vi "Teleop.vi"(10 "Match Info":T1={"Autonomous Elapsed Seconds"=0.0, "TeleOp Elapsed Seconds"=768.189, "Disabled Elapsed Seconds"=20.969, "Visited Autonomous"=FALSE, "Visited TeleOp"=TRUE, "Visited Disabled"=TRUE, "Autonomous Settings"={"Autonomous Style"=enum."Independent", "VI Refnum"=refnum}}, 11 "Call Context":T2=enum."Stop") -> ()   [LabVIEW 2020]
doc: "This VI is called for each TeleOp packet received from the DS where the robot is not disabled. It is often used to read from the joysticks and update I/O or to update setpoints for timed control loops. It should complete and return within 20 milliseconds or it may miss DS packets."
uses:
  <vilib>/Rock Robotics/WPI/DriverStation/WPI_DriverStationDerivedRobotMode.ctl
  <vilib>/Rock Robotics/WPI/DriverStation/WPI_DriverStationMatch Info.ctl
  <vilib>/Rock Robotics/Network Tables/NT Read Boolean.vi
  <vilib>/Rock Robotics/WPI/Utilities/WPI_GetSetVariantRefNum.vi
  <vilib>/Rock Robotics/Network Tables/NT Write Numeric Array.vi
  <vilib>/Rock Robotics/Network Tables/NT Write Boolean Array.vi
  <vilib>/Rock Robotics/Network Tables/NT Write Boolean.vi
  <vilib>/Rock Robotics/Network Tables/NT Read Number.vi
  Robot Global Data.vi
  <vilib>/Rock Robotics/WPI/ThirdParty/Phoenix-LabVIEW/Motor Controller/Controls/CTRE_Phoenix_MotorControl_ControlMode.ctl
  <vilib>/Rock Robotics/Network Tables/NT Write Number.vi
panel:
  out "Sample Boolean 0":bool
  out "Sample Slider 0":dbl(slide) scale=0.0..5.0
  out "Sample Boolean 2":bool
  out "Sample Slider 2":dbl(slide) scale=0.0..5.0
  out "Sample Boolean 1":bool
  out "Sample Slider1":dbl(slide) scale=0.0..5.0
  in  "Joysticks":u16(ring) items=["RIGHT TANK (default)", "LEFT ARM", "RIGHT ARM", "LEFT TANK DRIVE"]
  in  "AXIS VALUES":u16(ring) items=["X axis", "Y axis", "Z axis"]
  in  "NORMAL":cluster{"button":i32, "%speed":dbl}={"button"=0, "%speed"=0.75} {"%speed" min=0.0 max=1.0 format="%.3g"}
  in  "TURTLE":cluster{"button":i32, "%speed":dbl}={"button"=4, "%speed"=0.5} {"%speed" min=0.0 max=1.0 format="%.3g"}
  in  "TURBO":cluster{"button":i32, "%speed":dbl}={"button"=2, "%speed"=1.0} {"%speed" min=0.0 max=1.0 format="%.3g"}
  # "JOYSTICK 1  (left drive)\nBUTTONS & CONTROLS\n\nBTN 0 - BUMP INTAKE \nBTN 1 - FORCE INTAKE down\nBTN 2 -  \nBTN 3 - \nBTN 4 - \nBTN 5 - \nBTN 6 - \n\nPOV - \n\nX - \nY - drive LEFT forward/reverse\nZ -\nROT -"
  # "JOYSTICK 0  (right drive)\nBUTTONS & CONTROLS\n\nBTN 0 - FIRE cargo\nBTN 1 - TURBO drive \nBTN 2 - \nBTN 3 - \nBTN 4 - \nBTN 5 - TURTLE drive\nBTN 6 - RE-CENTER POV camera\n\nPOV - camera servo?\n\nX - drive left/right\nY - drive RIGHT forward/reverse\nZ -\nROT -"
  # "JOYSTICK LEFT  arm\nBUTTONS & CONTROLS\n\nX - left rotate arm forward\nY - forward raises climber\n\nBTN  7 - OVERIDE PGM\nBTN  8 - MACRO FWD\nBTN  9 - MACRO REV \nBTN 10 - TOGGLE INTAKE UP/DN\nBTN 11 - INTAKE ROLLER TOGGLE\nBTN 12 - LOW CLIMB MACRO"
  # "JOYSTICK RIGHT  arm\nBUTTONS & CONTROLS\n\nX - left rotate arm forward\nY - forward raises climber\n\nBTN  7 - FIRE CARGO\nBTN  8 - SHOOTER HI speed\nBTN  9 - SHOOTER LO speed\nBTN 10 - \nBTN 11 - PUKE BALL\nBTN 12 - SHOOTER STOP"
  # "to START MOKEY BAR CLIMBING MACRO, PRESS & HOLD BTN 8 & 9"
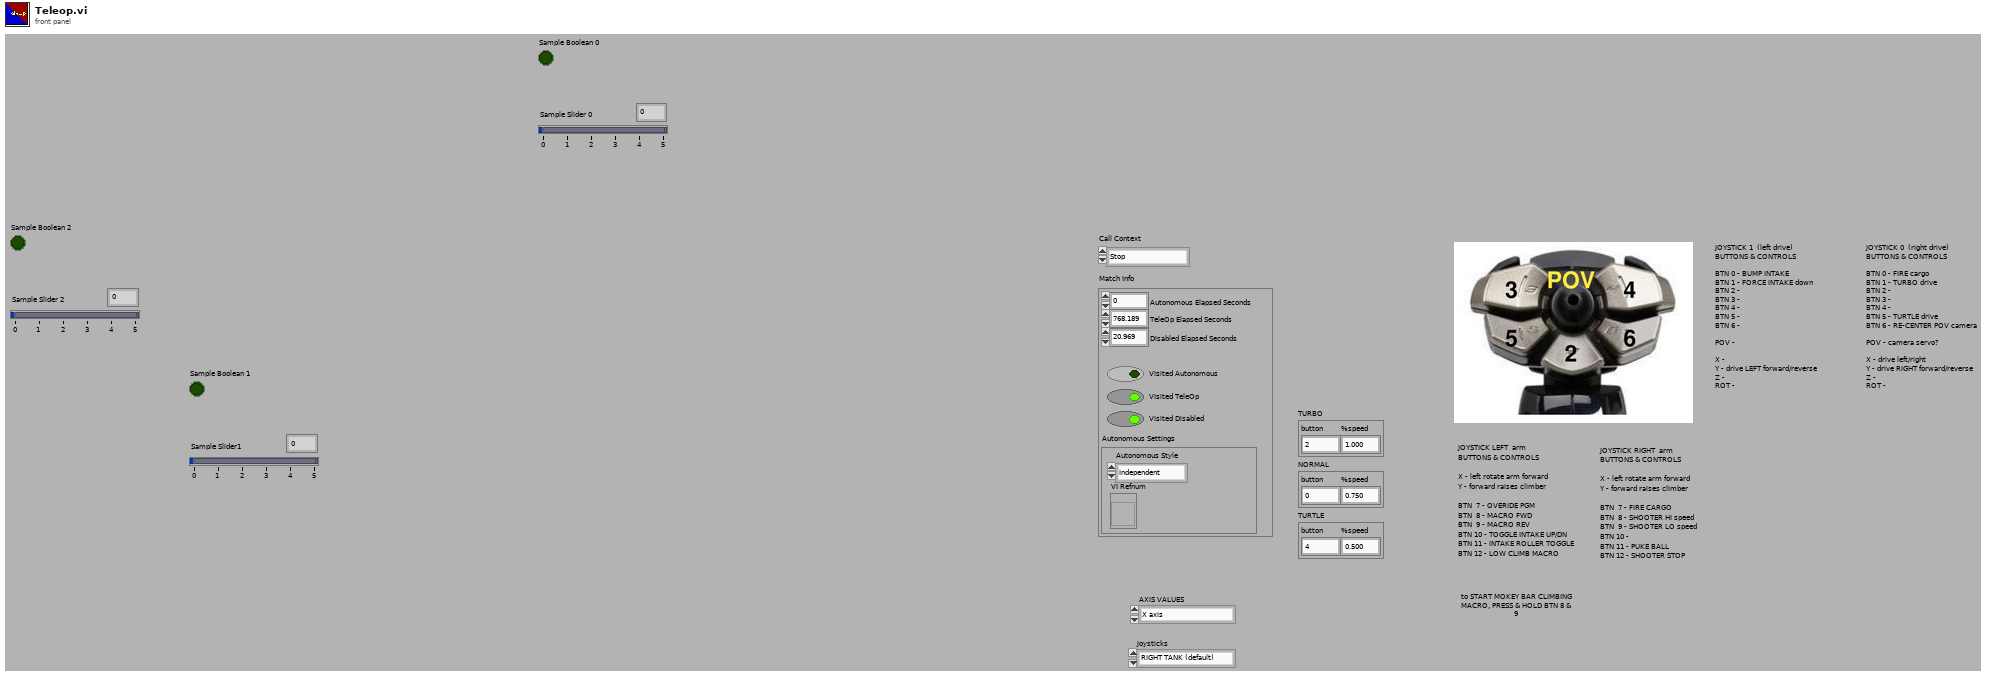
[diagram p1: front panel]
types:
  T1 = typedef "WPI_DriverStationMatch Info.ctl" = cluster{"Autonomous Elapsed Seconds":dbl, "TeleOp Elapsed Seconds":dbl, "Disabled Elapsed Seconds":dbl, "Visited Autonomous":bool, "Visited TeleOp":bool, "Visited Disabled":bool, "Autonomous Settings":cluster{"Autonomous Style":enum16{"Iterative", "Independent"}, "VI Refnum":refnum<vi>}}
  T2 = typedef "WPI_DriverStationDerivedRobotMode.ctl" = enum16{"Init", "Execute", "Stop"}
  T3 = typedef "CTRE_Phoenix_MotorControl_ControlMode.ctl" = u16
  T4 = typedef "WPI_MotorControlDeviceRef.ctl" = cluster{"DeviceStatus":errorcluster, "Type":T5, "PWM":cluster{"PWM Channel":T6, "DeadBand":T7}, "CAN":cluster{"Device Number":u8, "SetOutput VI Ref":variant, "GetOutput VI Ref":variant, "Enable VI Ref":variant, "Disable VI Ref":variant, "Data":variant}, "Invert":bool, "DIO PWM":cluster{"PWM \"Enable\" Channel":T6, "DIOChannel":T8, "PWM Rate":dbl}}
  T5 = typedef "WPI_MotorControlType.ctl" = enum16{"PWM", "CAN", "DIO PWM"}
  T6 = typedef "FPGA_DIOPWMChannel.ctl" = enum8{"PWM 0", "PWM 1", "PWM 2", "PWM 3", "PWM 4", "PWM 5", "PWM 6", "PWM 7", "PWM 8", "PWM 9", "PWM MXP 0", "PWM MXP 1", "PWM MXP 2", "PWM MXP 3", "PWM MXP 4", "PWM MXP 5", "PWM MXP 6", "PWM MXP 7", "PWM MXP 8", "PWM MXP 9", "Invalid"}
  T7 = typedef "WPI_PWMDeadband.ctl" = cluster{"Name":string, "maxPositivePwm":i32, "minPositivePwm":i32, "centerPwm":i32, "maxNegativePwm":i32, "minNegativePwm":i32, "angularRange":u16}
  T8 = typedef "FPGA_DIOChannel.ctl" = enum8{"DIO 0", "DIO 1", "DIO 2", "DIO 3", "DIO 4", "DIO 5", "DIO 6", "DIO 7", "DIO 8", "DIO 9", "DIO MXP 0", "DIO MXP 1", "DIO MXP 2", "DIO MXP 3", "DIO MXP 4", "DIO MXP 5", "DIO MXP 6", "DIO MXP 7", "DIO MXP 8", "DIO MXP 9", "DIO MXP 10", "DIO MXP 11", "DIO MXP 12", "DIO MXP 13", "DIO MXP 14", "DIO MXP 15", "SPI Port CS1", "SPI Port CS2", "SPI Port CS3", "SPI Port MISO", "SPI Port MOSI", "Invalid"}
  T9 = cluster{"MIN":dbl, "MAX":dbl, "convert climber inches to tics":dbl, "INITIALIZE":dbl}
  T10 = typedef "WPI_JoystickDevRef.ctl" = cluster{"Device":T11}
  T11 = typedef "WPI_JoystickDeviceEnum.ctl" = enum16{"USB 0", "USB 1", "USB 2", "USB 3", "USB 4", "USB 5"}
  T12 = cluster{"Axes":dbl[], "Buttons":bool[], "POVs":i16[]}[]
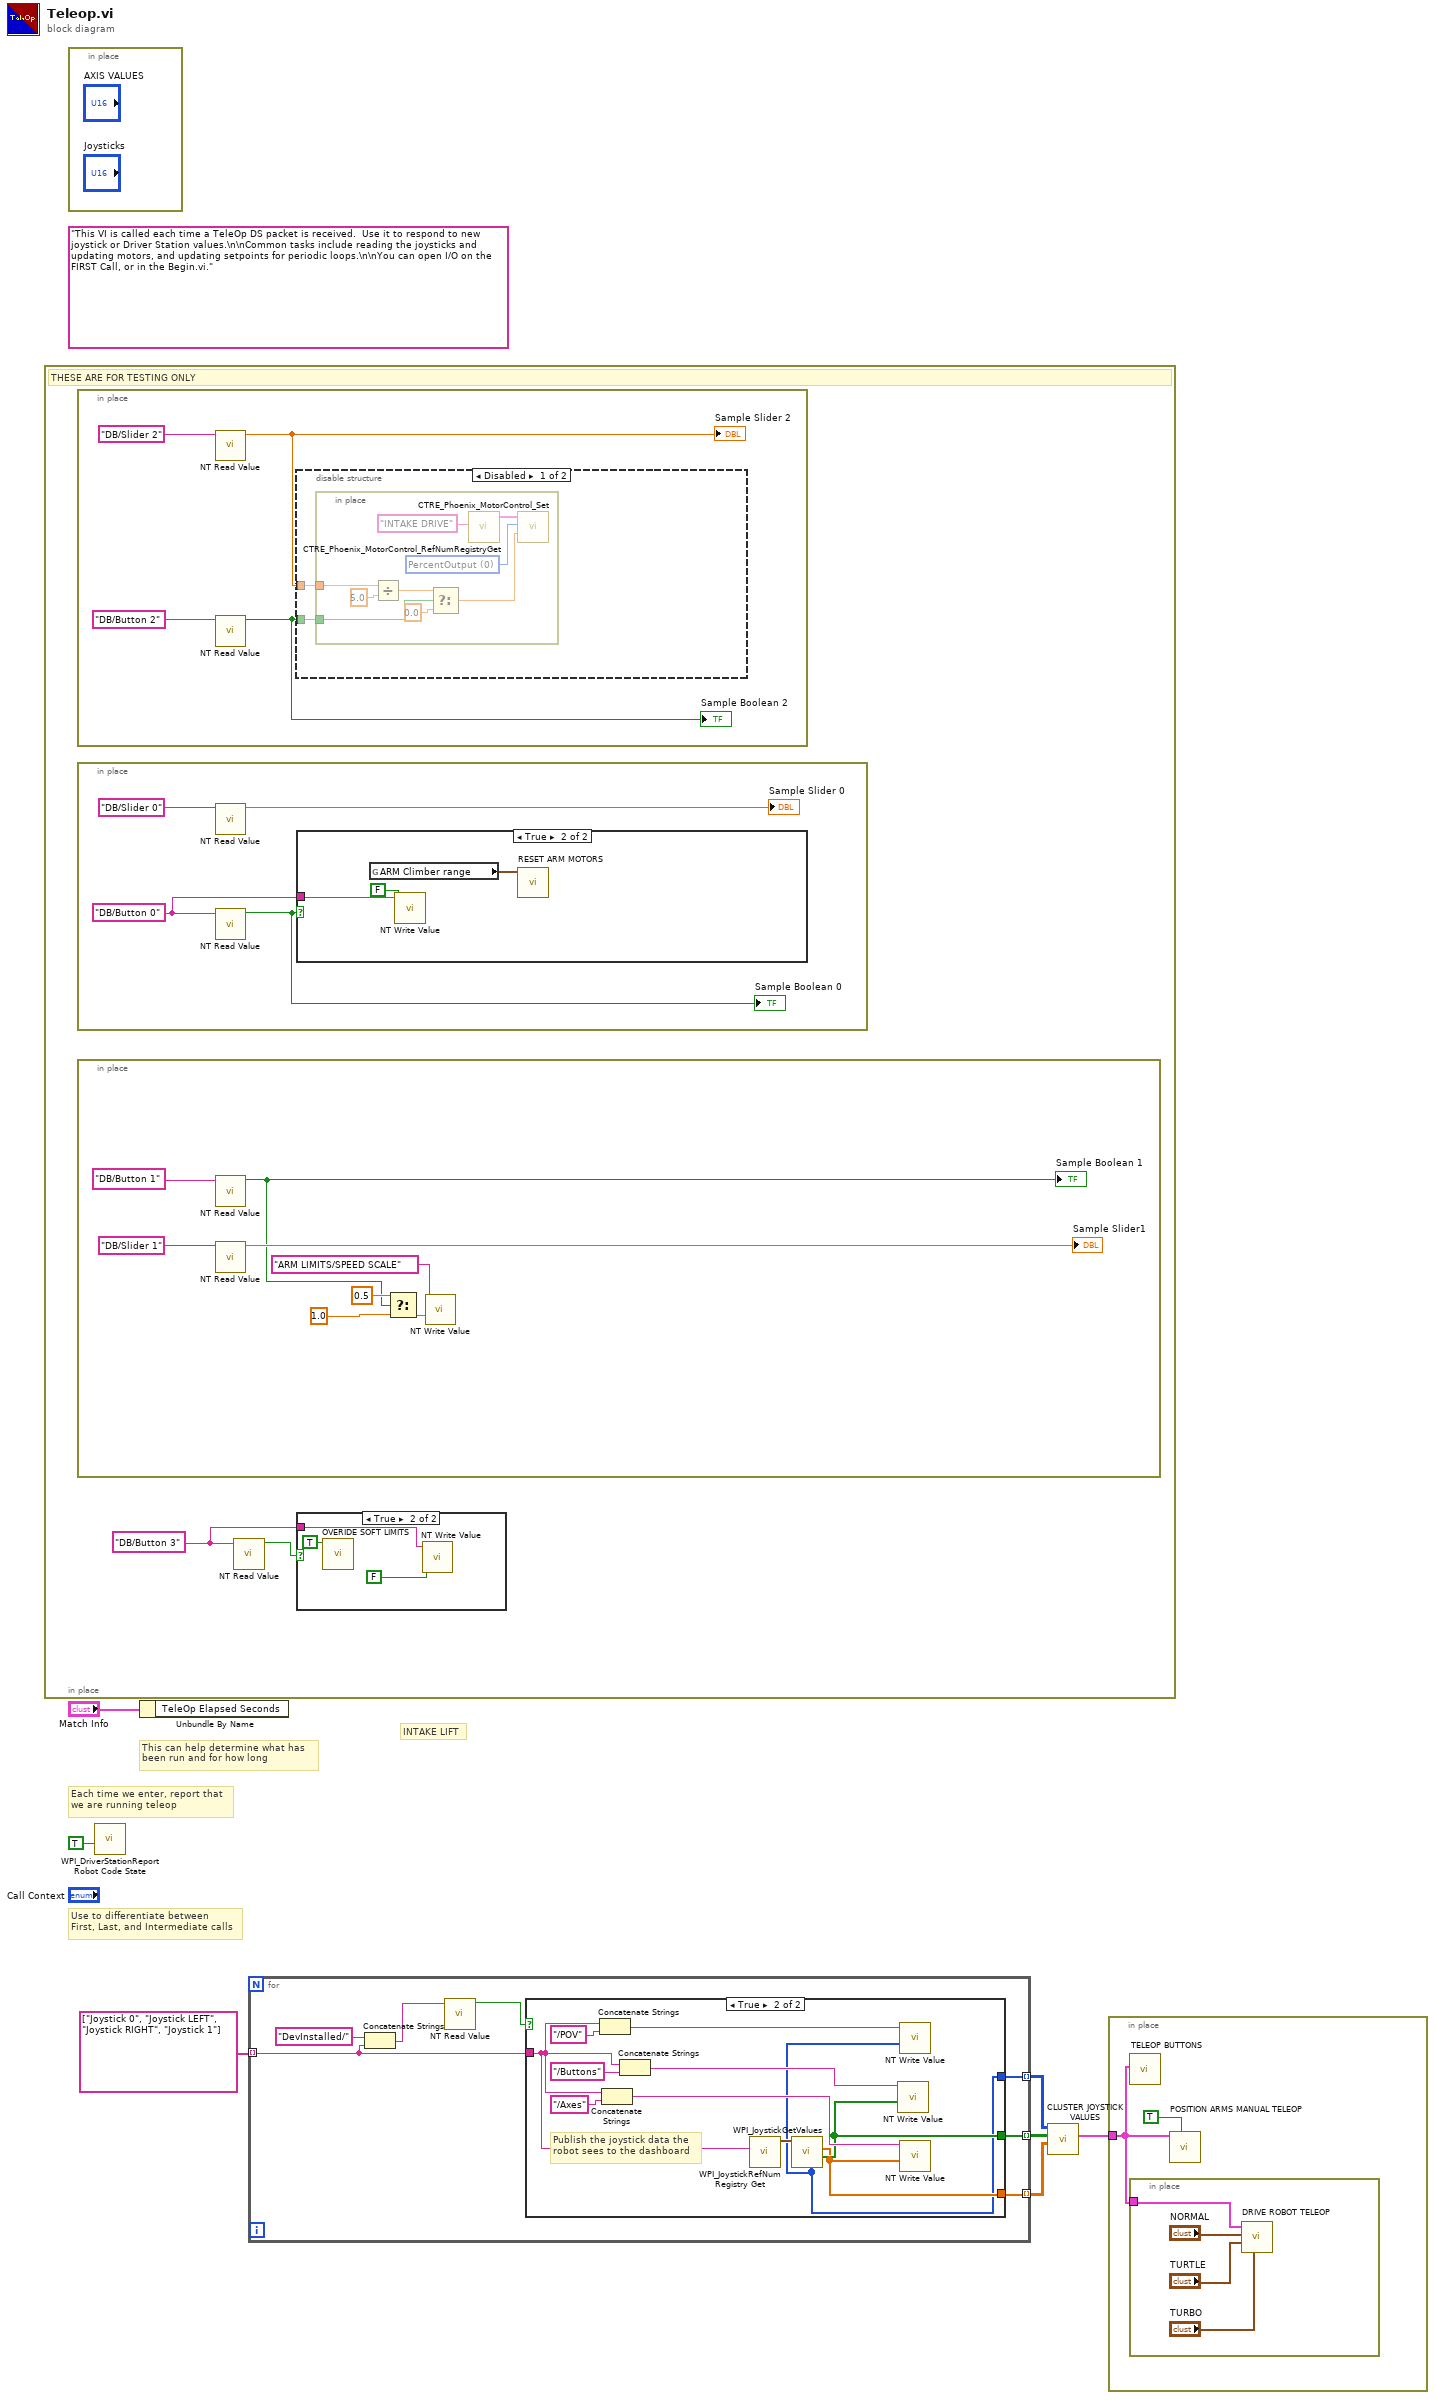
[diagram p0: block diagram]
diagram:
  (unwired) "This VI is called each time a TeleOp DS packet is received.  Use it to respond to new joystick or Driver Station values.\n\nCommon tasks include reading the joysticks and updating motors, and updating setpoints for periodic loops.\n\nYou can open I/O on the FIRST Call, or in the Begin.vi."
  # "INTAKE LIFT"
  # "Each time we enter, report that\nwe are running teleop"
  # "Use to differentiate between\nFirst, Last, and Intermediate calls"
  # "This can help determine what has\nbeen run and for how long"
  n1 = in-place {
    w8 = "DB/Button 3" ("refnum name")
    # "THESE ARE FOR TESTING ONLY"
    n2 = in-place {
      n3 = call-poly <vilib>:"NT Read Value.vi"("Name"="DB/Slider 2" ("refnum name")) -> ("Numeric"=w21:dbl)  [unwired: 9 in, 1 out]
      "Sample Slider 2" <- w21
      n4 = call-poly <vilib>:"NT Read Value.vi"("Name"="DB/Button 2" ("refnum name")) -> ("Boolean"=w20:bool)  [unwired: 9 in, 1 out]
      "Sample Boolean 2" <- w20
      n5 = disable-structure shown="Disabled" {
        disable-tunnel: w21 -> [w25 _]
        disable-tunnel: w20 -> [w24 _]
        frame Disabled {
          n6 = in-place {
            in-place-border: w25 -> [w34]
            in-place-border: w24 -> [w28]
            w31 = T3 0 items=["PercentOutput"=0, "Position"=1, "Velocity"=2, "Current"=3, "Follower"=5, "MotionProfile"=6, "MotionMagic"=7, "MotionProfileArc"=10, "Disabled"=15] ("Control Mode")
            n7 = Divide(x=w34, y=5.0) -> (x/y=w27:dbl)
            n8 = Select(t=w27, s=w28, f=0.0) -> (s? t:f=w29:dbl)
            n9 = call <vilib>:"CTRE_Phoenix_MotorControl_RefNumRegistryGet.vi"("refnum name"="INTAKE DRIVE") -> ("PhoenixMotorControlDevRef"=w32:T4)  [unwired: 9 in, 1 out]
            n10 = call <vilib>:"CTRE_Phoenix_MotorControl_Set.vi"("Output"=w29, "Control Mode"=w31, "PhoenixMotorControlDevRef"=w32) -> ()  [unwired: 7 in, 2 out]
          }
        }
        frame Enabled {
        }
      }
    }
    n11 = in-place {
      w13 = "DB/Button 0" ("refnum name")
      n12 = call-poly <vilib>:"NT Read Value.vi"("Name"="DB/Slider 0" ("refnum name")) -> ("Numeric"=→"Sample Slider 0":dbl)  [unwired: 9 in, 1 out]
      n13 = call-poly <vilib>:"NT Read Value.vi"("Name"=w13) -> ("Boolean"=w14:bool)  [unwired: 9 in, 1 out]
      "Sample Boolean 0" <- w14
      n14 = case shown="True" w14 {
        tunnel: w13 -> [_ w19]
        frame False {
        }
        frame True {
          n15 = global read "Robot Global Data.vi" "ARM Climber range"() -> (w18:T9)
          n16 = call-poly <vilib>:"NT Write Value.vi"("Boolean"=FALSE, "Name"=w19) -> ()  [unwired: 9 in, 1 out]
          n17 = call "RESET ARM MOTORS.vi"("ARM Climber range"=w18) -> ()  [unwired: 8 in, 3 out]
        }
      }
    }
    n18 = in-place {
      n19 = call-poly <vilib>:"NT Read Value.vi"("Name"="DB/Button 1" ("refnum name")) -> ("Boolean"=w35:bool)  [unwired: 9 in, 1 out]
      "Sample Boolean 1" <- w35
      n20 = call-poly <vilib>:"NT Read Value.vi"("Name"="DB/Slider 1" ("refnum name")) -> ("Numeric"=→"Sample Slider1":dbl)  [unwired: 9 in, 1 out]
      n21 = Select(t=0.5, s=w35, f=1.0 ("Numeric")) -> (s? t:f=w37:dbl)
      n22 = call-poly <vilib>:"NT Write Value.vi"("Numeric"=w37, "Name"="ARM LIMITS/SPEED SCALE") -> ()  [unwired: 9 in, 1 out]
    }
    n23 = call-poly <vilib>:"NT Read Value.vi"("Name"=w8) -> ("Boolean"=w9:bool)  [unwired: 9 in, 1 out]
    n24 = case shown="True" w9 {
      tunnel: w8 -> [_ w11]
      frame False {
      }
      frame True {
        n25 = call "OVERIDE SOFT LIMITS.vi"("Override Limit Switches?"=TRUE) -> ()  [unwired: 11 in]
        n26 = call-poly <vilib>:"NT Write Value.vi"("Boolean"=FALSE, "Name"=w11) -> ()  [unwired: 9 in, 1 out]
      }
    }
  }
  n27 = in-place {
  }
  n28 = call <vilib>:"WPI_DriverStationReport Robot Code State.vi"("TeleOp"=TRUE ("Autonomous")) -> ()  [unwired: 10 in, 1 out]
  n29 = Unbundle By Name("Match Info") -> ()  [unwired: 1 out]
  n30 = for {
    tunnel: string[] ["Joystick 0", "Joystick LEFT", "Joystick RIGHT", "Joystick 1"] -> [w46] mode=indexing
    tunnel: [w44] -> w2 mode=indexing
    tunnel: [w45] -> w3 mode=indexing
    tunnel: [w43] -> w1 mode=indexing
    n31 = Concatenate Strings("DevInstalled/" ("string"), w46) -> (w48:string)
    n32 = call-poly <vilib>:"NT Read Value.vi"("Name"=w48) -> ("Boolean"=w47:bool)  [unwired: 9 in, 1 out]
    n33 = case shown="True" w47 {
      tunnel: w46 -> [_ w53]
      tunnel: [_ w52] -> w44
      tunnel: [_ w51] -> w45
      tunnel: [_ w50] -> w43
      frame False {
      }
      frame True {
        # "Publish the joystick data the\nrobot sees to the dashboard"
        n34 = Concatenate Strings(w53, "/POV" ("Name")) -> (w55:string)
        n35 = Concatenate Strings(w53, "/Axes" ("Name")) -> (w54:string)
        n36 = Concatenate Strings(w53, "/Buttons" ("Name")) -> (w56:string)
        n37 = call <vilib>:"WPI_JoystickRefNum Registry Get.vi"("refnum name"=w53) -> ("JoystickDevRef"=w60:T10)  [unwired: 1 in, 9 out]
        n38 = call <vilib>:"WPI_JoystickGetValues.vi"("JoystickDevRef"=w60) -> ("Buttons"=w52:bool[], "Axes"=w51:dbl[], "POVs"=w50:i16[])  [unwired: 6 in, 2 out]
        n39 = call-poly <vilib>:"NT Write Value.vi"("Boolean Array"=w52, "Name"=w56) -> ()  [unwired: 9 in, 1 out]
        n40 = call-poly <vilib>:"NT Write Value.vi"("Numeric Array"=w50, "Name"=w55) -> ()  [unwired: 9 in, 1 out]
        n41 = call-poly <vilib>:"NT Write Value.vi"("Numeric Array"=w51, "Name"=w54) -> ()  [unwired: 9 in, 1 out]
      }
    }
  }
  n42 = call "CLUSTER JOYSTICK VALUES.vi"("Axes"=w3, "Buttons"=w2, "POVs"=w1) -> ("Joystick values"=w7:T12)  [unwired: 8 in]
  n43 = in-place {
    in-place-border: w7 -> [w62]
    n44 = call "TELEOP BUTTONS.vi"("Joystick values"=w62) -> ()  [unwired: 11 in]
    n45 = in-place {
      in-place-border: w62 -> [w66]
      n46 = call "DRIVE ROBOT TELEOP.vi"("TURBO"="TURBO", "TURTLE"="TURTLE", "NORMAL"="NORMAL", "Joystick values"=w66) -> ()  [unwired: 8 in]
    }
    n47 = call "POSITION ARMS MANUAL TELEOP.vi"("Use percent output?"=TRUE, "Joystick values"=w62) -> ()  [unwired: 10 in]
  }
